vi "select multiple files.vi"() -> ()   [LabVIEW 2025]
uses:
  <vilib>/Utility/file.llb/Read Delimited Spreadsheet (DBL).vi
panel:
  in  "stop":bool
  out "selected path":path[](array[path])
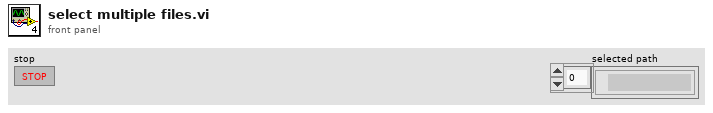
[diagram p1: front panel]
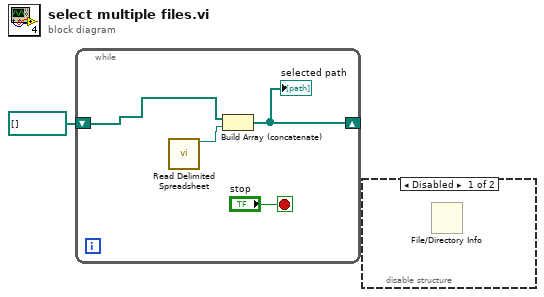
[diagram p0: block diagram]
diagram:
  n1 = while {
    shift-right: [w2] -> _
    shift-left: path[] [] -> [w5]
    stop <- "stop" stop-if-true
    n2 = call-poly <vilib>:"Read Delimited Spreadsheet.vi"() -> ("new file path (Not A Path if cancelled)"=w3:path)  [unwired: 10 in, 5 out]
    n3 = Build Array (concatenate)(w5, w3) -> (w2:path[])
    "selected path" <- w2
  }
  n4 = disable-structure shown="Disabled" {
    frame Disabled {
      n5 = File/Directory Info() -> ()  [unwired: 2 in, 7 out]
    }
    frame Enabled {
    }
  }
